vi "调整采样率.vi"(3 "目标采样率 Hz":u8, 4 "输入":T1(array[cluster])) -> (1 "输出":T1(array[cluster]))   [LabVIEW 2017]
panel:
  out "接收到x组数据":i32
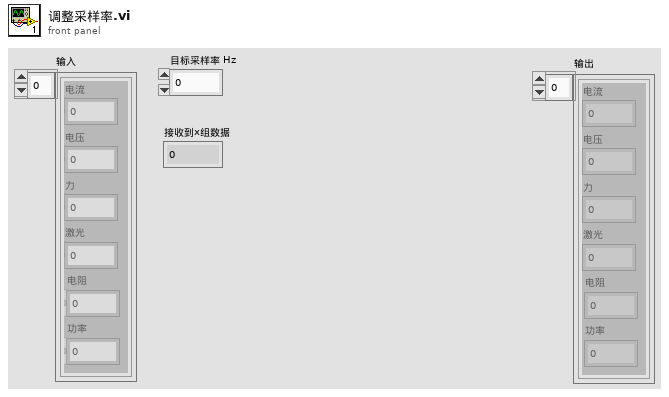
[diagram p1: front panel]
types:
  T1 = cluster{"电流":dbl, "电压":dbl, "力":dbl, "激光":dbl, "电阻":dbl, "功率":dbl}[]
  T2 = cluster{"电流":dbl, "电压":dbl, "力":dbl, "激光":dbl, "电阻":dbl, "功率":dbl}
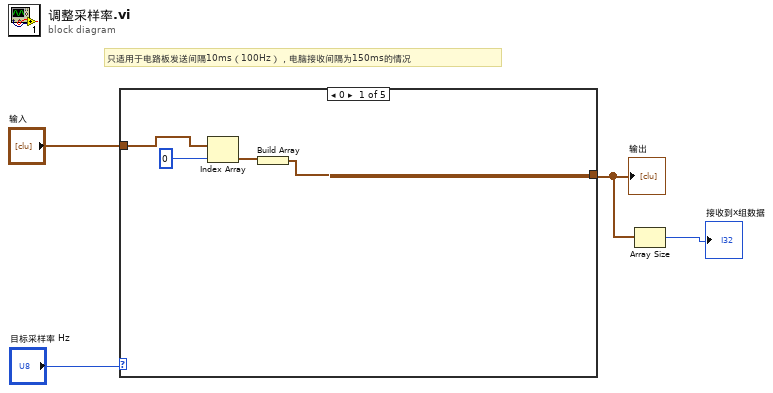
[diagram p0: block diagram]
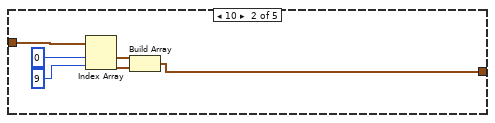
[diagram p2: hidden frame]
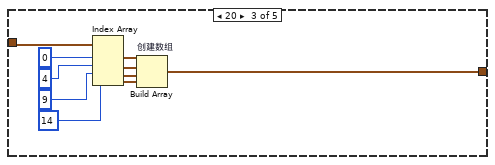
[diagram p3: hidden frame]
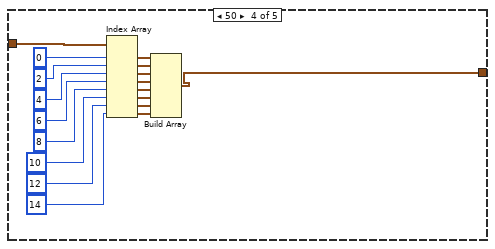
[diagram p4: hidden frame]
diagram:
  # "只适用于电路板发送间隔10ms（100Hz），电脑接收间隔为150ms的情况"
  n1 = case shown="0" "目标采样率 Hz" {
    tunnel: "输入" -> [w6 w10 w16 w26 w43]
    tunnel: [w5 w9 w15 w25 w43] -> w2
    frame 0 {
      n2 = Index Array(array=w6, index=0) -> (element=w8:T2)
      n3 = Build Array(w8) -> (w5:T1)
    }
    frame 10 {
      n4 = Index Array(array=w10, index #1=0, index #2=9) -> (element #1=w13:T2, element #2=w14:T2)
      n5 = Build Array(w13, w14) -> (w9:T1)
    }
    frame 20 {
      n6 = Index Array(array=w16, index #1=0, index #2=4, index #3=9, index #4=14) -> (element #1=w24:T2, element #2=w23:T2, element #3=w22:T2, element #4=w21:T2)
      n7 = Build Array "创建数组"(w24, w23, w22, w21) -> (w15:T1)
    }
    frame 50 {
      n8 = Index Array(array=w26, index #1=0, index #2=2, index #3=4, index #4=6, index #5=8, index #6=10, index #7=12, index #8=14) -> (element #1=w38:T2, element #2=w37:T2, element #3=w36:T2, element #4=w35:T2, element #5=w39:T2, element #6=w40:T2, element #7=w41:T2, element #8=w42:T2)
      n9 = Build Array(w38, w37, w36, w35, w39, w40, w41, w42) -> (w25:T1)
    }
    frame 100, Default {
    }
  }
  "输出" <- w2
  n10 = Array Size(array=w2) -> (size(s)=→"接收到x组数据":i32)
